vi "Simple AAP.vi"() -> ()   [LabVIEW 2014]
panel:
  out "Average Value":dbl
  out "Waveform Graph":dynamicdata(graph)
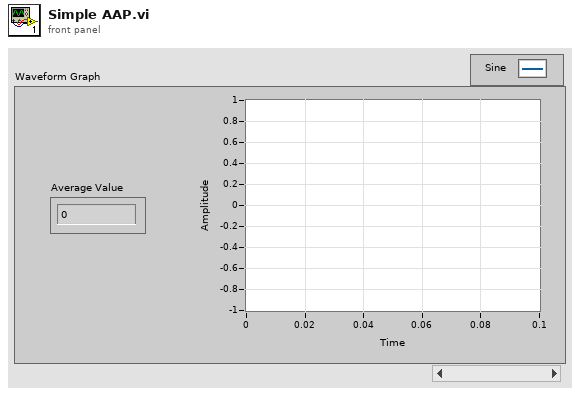
[diagram p1: front panel]
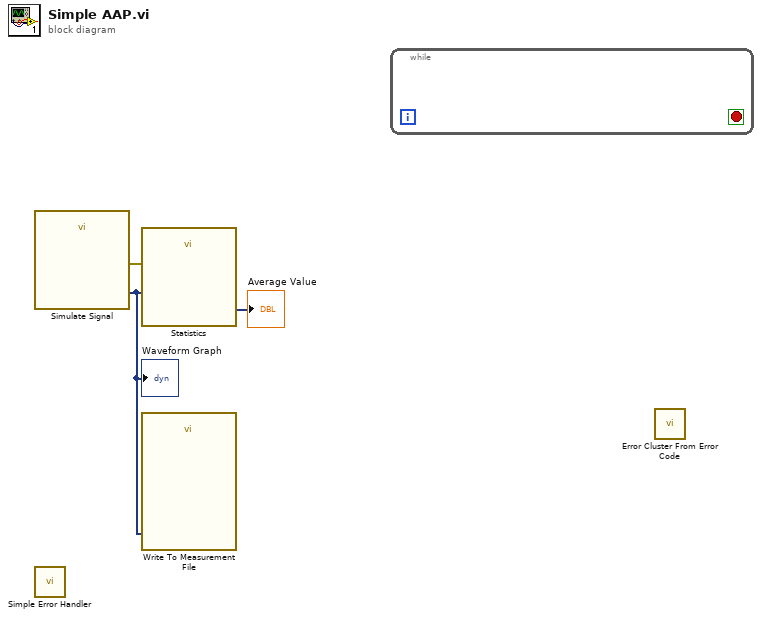
[diagram p0: block diagram]
diagram:
  n1 = call "Simulate Signal"() -> ("Sine"=w2:dynamicdata, "error out"=w1:errorcluster)  [unwired: 14 in]
  "Waveform Graph" <- w2
  n2 = call <vilib>:"Simple Error Handler.vi"() -> ()  [unwired: 5 in, 5 out]
  n3 = call "Statistics"("Signals"=w2, "error in (no error)"=w1) -> ("Arithmetic Mean"=→"Average Value":dynamicdata)  [unwired: 24 in, 1 out]
  n4 = call "Write To Measurement File"("Signals"=w2) -> ()  [unwired: 16 in, 3 out]
  n5 = while {
    stop <- _ stop-if-true
  }
  n6 = call <vilib>:"Error Cluster From Error Code.vi"() -> ()  [unwired: 9 in, 1 out]
